vi "Errorbar2003.vi"   [LabVIEW 2013]
uses:
  ModeType.ctl
  <vilib>/Heliosphere Research LLC/Advanced Plotting Toolkit/Advanced Plotting Toolkit.lvlib
types:
  T1 = typedef "ModeType.ctl" = enum16{"Normal", "Expected Failure", "Skipped", "Broken"}
  T2 = typedef "Advanced Plotting Toolkit.lvlib/PlotID.ctl" = i32
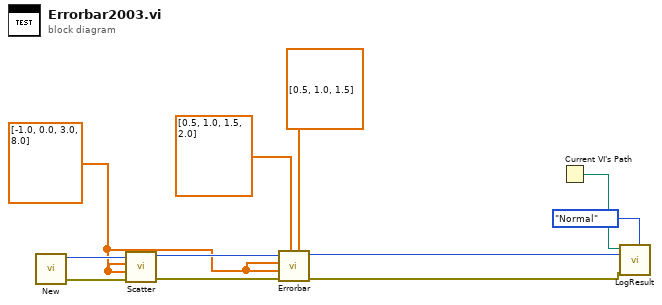
[diagram p0: block diagram]
diagram:
  w4 = dbl[] [-1.0, 0.0, 3.0, 8.0] ("X Data")
  n1 = call <vilib>:"New.vi"() -> ("error out"=w5:errorcluster, "Plot ID"=w8:T2)  [unwired: 10 in]
  n2 = call <vilib>:"Scatter.vi"("error in (no error)"=w5, "Y Data"=w4, "X Data"=w4, "Plot ID"=w8) -> ("error out"=w6:errorcluster, "Plot ID Out"=w7:T2)  [unwired: 6 in]
  n3 = call <vilib>:"Errorbar.vi"("Y Errors"=dbl[] [0.5, 1.0, 1.5] ("X Errors"), "X Errors"=dbl[] [0.5, 1.0, 1.5, 2.0], "error in (no error)"=w6, "Y Data"=w4, "X Data"=w4, "Plot ID"=w7) -> ("error out"=w9:errorcluster, "Plot ID out"=w10:T2)  [unwired: 4 in]
  n4 = Current VI's Path() -> (path=w11:path)
  n5 = call "LogResult.vi"("Mode"=ModeType."Normal", "Test Result"=w9, "Test Artifact"=w10, "VI Path"=w11) -> ()  [unwired: 8 in]
